vi "Calibration - Data (FGV).vi"(7 "Action":T2=enum."Write", 8 "error In":errorcluster, 11 "Calib":T1={"Timeout"=-1, "LC MC"=[], "TD MC"=[], "Motor Pulse"=0, "Disp M"=[], "LC Unit"=[], "Disp Unit"=[], "TD Unit"=[], "LC Name"=[], "TD Name"=[], "Machine"=enum."Please Select", "Sensor Port"=[]}) -> (0 "error out":errorcluster, 3 "Calib out":T1={"Timeout"=-1, "LC MC"=[], "TD MC"=[], "Motor Pulse"=0, "Disp M"=[], "LC Unit"=[], "Disp Unit"=[], "TD Unit"=[], "LC Name"=[], "TD Name"=[], "Machine"=enum."Please Select", "Sensor Port"=[]})   [LabVIEW 2019]
uses:
  Controls/FGV States.ctl
  Controls/Calibration - Data Structure.ctl
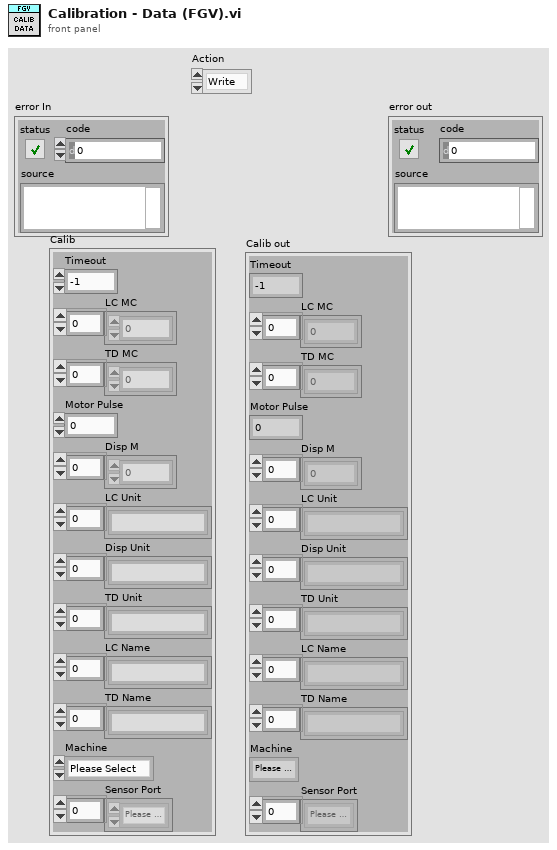
[diagram p1: front panel]
types:
  T1 = typedef "Calibration - Data Structure.ctl" = cluster{"Timeout":i32, "LC MC":dbl[], "TD MC":dbl[], "Motor Pulse":u64, "Disp M":dbl[], "LC Unit":string[], "Disp Unit":string[], "TD Unit":string[], "LC Name":string[], "TD Name":string[], "Machine":enum16{"Please Select", "Motor 1", "Motor 2", "Motor 3", "Motor 4", "Motor 5", "Motor 6", "Motor 7", "Motor 8", "Motor 9"}, "Sensor Port":enum16{"Please Select", "LC 1", "LC 2", "LC 3", "LC 4", "LC 5", "LC 6", "LC 7", "LC 8", "TD 1", "TD 2", "TD 3", "TD 4", "TD 5", "TD 6", "TD 7", "TD 8", "TD 9", "TD 10", "TD 11", "TD 12"}[]}
  T2 = typedef "FGV States.ctl" = enum16{"Read", "Write"}
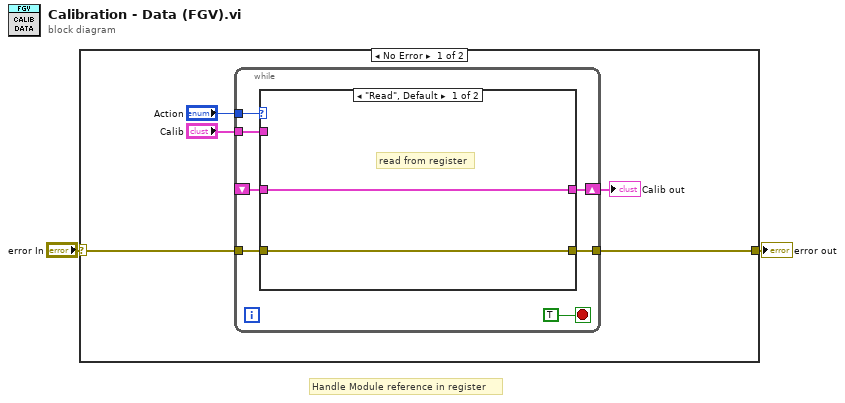
[diagram p0: block diagram]
diagram:
  # "Handle Module reference in register"
  n1 = case shown="No Error" "error In" {
    selector: "error In" -> [w6 w19]
    tunnel: [w5 w19] -> w1
    frame No Error {
      n2 = while {
        tunnel: "Action" -> [w14]
        tunnel: "Calib" -> [w11]
        shift-right: [w12] -> w3
        shift-left: _ -> [w10]
        tunnel: [w9] -> w5
        tunnel: w6 -> [w8]
        stop <- TRUE stop-if-true
        n3 = case shown="\"Read\", Default" w14 {
          tunnel: [w15 w18] -> w12
          tunnel: w11 -> [_ w18]
          tunnel: w10 -> [w15 _]
          tunnel: [w16 w17] -> w9
          tunnel: w8 -> [w16 w17]
          frame "Read", Default {
            # "read from register"
          }
          frame "Write" {
            # "write to register"
          }
        }
      }
      "Calib out" <- w3
    }
    frame Error {
    }
  }
  "error out" <- w1
